vi "ExSubCloseMult.vi"(1 "error in (no error)":errorcluster, 2 "Handles In":T1) -> (0 "error out":errorcluster)   [LabVIEW 2010]
panel:
  # "ExSubCloseMult:\nThis sub vi closes the multiple camera experiment."
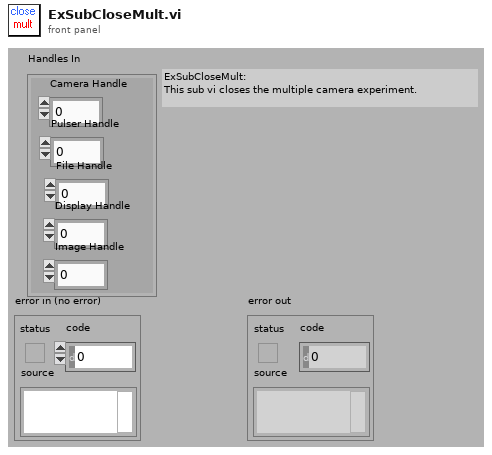
[diagram p1: front panel]
types:
  T1 = cluster{"Camera Handle":u32, "Pulser Handle":u32, "File Handle":u32, "Display Handle":u32, "Image Handle":u32}
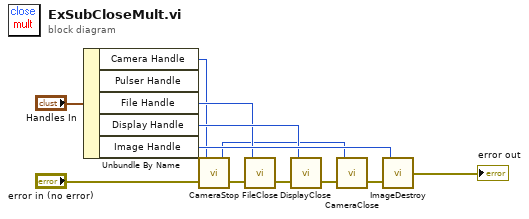
[diagram p0: block diagram]
diagram:
  n1 = Unbundle By Name("Handles In") -> ("Camera Handle"=w2:u32, "File Handle"=w8:u32, "Display Handle"=w9:u32, "Image Handle"=w10:u32)  [unwired: 1 out]
  n2 = call <userlib>:"CameraStop.vi"("error in"="error in (no error)", "Camera Handle"=w2) -> ("error out"=w6:errorcluster, "Camera Handle"=w7:u32)
  n3 = call <userlib>:"FileClose.vi"("error in"=w6, "File Handle"=w8) -> ("error out"=w11:errorcluster)
  n4 = call <userlib>:"DisplayClose.vi"("error in"=w11, "Display Handle"=w9) -> ("error out"=w4:errorcluster)
  n5 = call <userlib>:"CameraClose.vi"("error in"=w4, "Camera Handle"=w7) -> ("error out"=w3:errorcluster)
  n6 = call <userlib>:"ImageDestroy.vi"("error in"=w3, "Data handle"=w10) -> ("error out"=→"error out":errorcluster)
